vi "FindReport (SubVI).vi"(8 "error in (no error)":errorcluster, 11 "ReportID":string) -> (0 "error out":errorcluster, 3 "Report path":path)   [LabVIEW 2018, in "MainFrameLib.lvlib"]
uses:
  MainFrameLib.lvlib
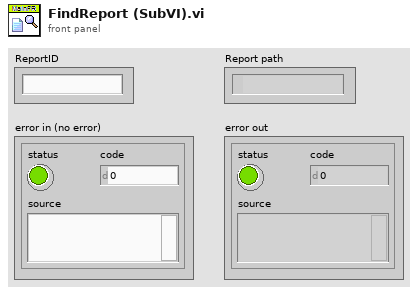
[diagram p1: front panel]
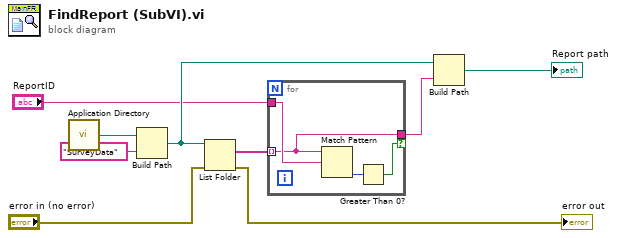
[diagram p0: block diagram]
diagram:
  n1 = call <vilib>:"Application Directory.vi"() -> ("Application Directory"=w1:path)
  n2 = Build Path(base path=w1, name or relative path="SurveyData") -> (appended path=w7:path)
  n3 = List Folder(path=w7, error in="error in (no error)") -> (filenames=w5:string[], error out=→"error out":errorcluster)  [unwired: 2 in, 2 out]
  n4 = for {
    tunnel: w5 -> [w11] mode=indexing
    tunnel: "ReportID" -> [w13]
    tunnel: [w11] -> w8 if=w10
    n5 = Match Pattern(string=w11, regular expression=w13) -> (offset past match=w12:i32)  [unwired: 1 in, 3 out]
    n6 = Greater Than 0?(x=w12) -> (x > 0?=w10:bool)
  }
  n7 = Build Path(base path=w7, name or relative path=w8) -> (appended path=→"Report path":path)
